vi "Read App.vi"(8 "error in (no error)":errorcluster, 10 "App Name":string, 11 "Path (*.ini)":path) -> (0 "error out":errorcluster, 3 "Name,Path,Section,VI,Group":string[][](array[string]))   [LabVIEW 2018, in "Shared.lvlib"]
uses:
  Shared.lvlib
  <vilib>/Utility/config.llb/NI_LVConfig.lvlib
  <vilib>/Utility/config.llb/Read Key (String).vi
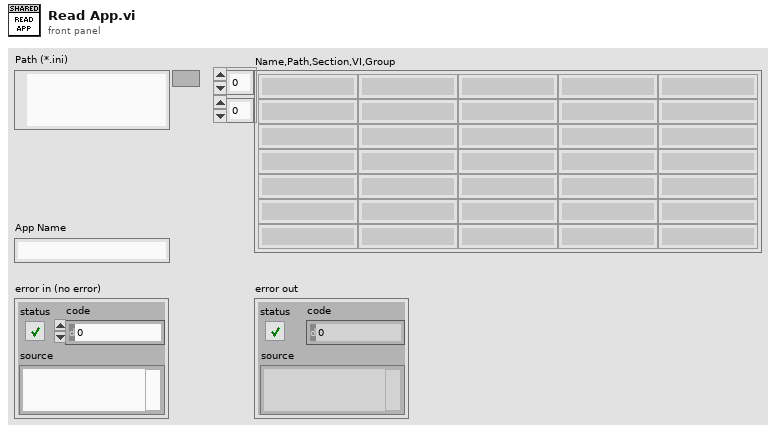
[diagram p1: front panel]
types:
  T1 = typedef "NI_LVConfig.lvlib/Config Data RefNum.ctl" = refnum<k1>
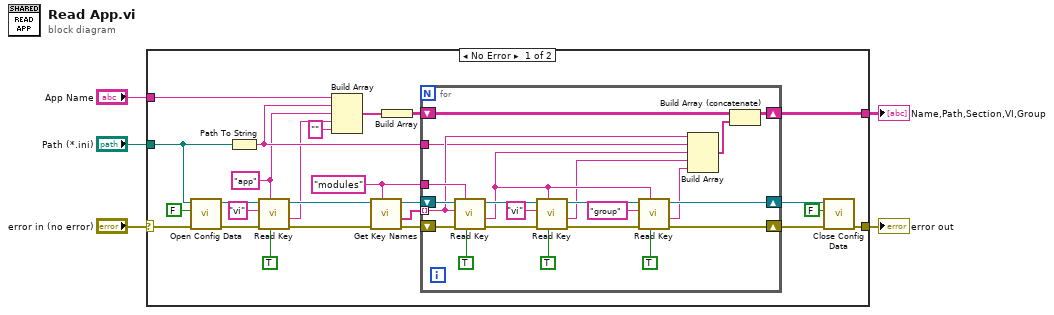
[diagram p0: block diagram]
diagram:
  n1 = case shown="No Error" "error in (no error)" {
    selector: "error in (no error)" -> [w8 w53]
    tunnel: "App Name" -> [w10 _]
    tunnel: "Path (*.ini)" -> [w9 _]
    tunnel: [w7 w53] -> w2
    tunnel: [w6 _] -> w1
    frame No Error {
      w15 = "app" ("section")
      w27 = "modules" ("section")
      n2 = call <vilib>:"Open Config Data.vi"("error in (no error)"=w8, "create file if necessary (T)"=FALSE, "configuration file path"=w9) -> ("error out"=w20:errorcluster, "refnum"=w21:T1)  [unwired: 6 in, 1 out]
      n3 = Path To String(path=w9) -> (string=w16:string)
      n4 = call-poly <vilib>:"Read Key.vi"("read raw string? (F)"=TRUE, "section"=w15, "error in (no error)"=w20, "key"="vi", "refnum"=w21) -> ("error out"=w19:errorcluster, "value"=w14:string, "refnum out"=w18:T1)  [unwired: 3 in, 1 out]
      n5 = Build Array(w10, w16, w15, w14, "" ("element")) -> (w12:string[])
      n6 = call <vilib>:"Get Key Names.vi"("section"=w27, "error in (no error)"=w19, "refnum"=w18) -> ("error out"=w24:errorcluster, "key names"=w28:string[], "refnum out"=w26:T1)  [unwired: 5 in, 1 out]
      n7 = Build Array(w12) -> (w11:string[][])
      n8 = for {
        shift-right: [w39] -> w25
        shift-left: w24 -> [w52]
        shift-right: [w40] -> w29
        shift-left: w26 -> [w51]
        tunnel: w27 -> [w49]
        tunnel: w28 -> [w37] mode=indexing
        tunnel: w16 -> [w34]
        shift-right: [w31] -> w6
        shift-left: w11 -> [w33]
        n9 = call-poly <vilib>:"Read Key.vi"("read raw string? (F)"=TRUE, "section"=w49, "error in (no error)"=w52, "key"=w37, "refnum"=w51) -> ("error out"=w46:errorcluster, "value"=w36:string, "refnum out"=w47:T1)  [unwired: 3 in, 1 out]
        n10 = call-poly <vilib>:"Read Key.vi"("read raw string? (F)"=TRUE, "section"=w36, "error in (no error)"=w46, "key"="vi", "refnum"=w47) -> ("error out"=w42:errorcluster, "value"=w35:string, "refnum out"=w41:T1)  [unwired: 3 in, 1 out]
        n11 = call-poly <vilib>:"Read Key.vi"("read raw string? (F)"=TRUE, "section"=w36, "error in (no error)"=w42, "key"="group", "refnum"=w41) -> ("error out"=w39:errorcluster, "value"=w38:string, "refnum out"=w40:T1)  [unwired: 3 in, 1 out]
        n12 = Build Array(w37, w34, w36, w35, w38) -> (w32:string[])
        n13 = Build Array (concatenate)(w33, w32) -> (w31:string[][])
      }
      n14 = call <vilib>:"Close Config Data.vi"("error in (no error)"=w25, "write file if changed (T)"=FALSE, "refnum"=w29) -> ("error out"=w7:errorcluster)  [unwired: 7 in, 1 out]
    }
    frame Error {
    }
  }
  "error out" <- w2
  "Name,Path,Section,VI,Group" <- w1
